vi "Image Difference RT Driver VI.vi"(10 "Device Outputs FIFO":refnum<k33>, 11 "Device Reference":T1 format="%.0x") -> ()   [LabVIEW 2012, in "Image Difference Custom Device.lvlib"]
uses:
  Image Difference Custom Device.lvlib
  <vilib>/NI Veristand/Custom Device API/Custom Device Item Ref.ctl
  <vilib>/NI Veristand/Custom Device API/Custom Device Channel Type.ctl
  <vilib>/NI Veristand/Custom Device API/Custom Device API.lvlib
  <vilib>/NI Veristand/Custom Device Tools/Custom Device Utility Library/Custom Device Utility Library.lvlib
  <vilib>/vision/driver/NI_Vision_Acquisition_Software.lvlib
panel:
  in  "Status Notifier":refnum<notifier>
  # "Custom Device Template\nv1.0"
  # "Use this template as a starting point for creating a custom device code module. The input controls shown here are specially named controls that the system will use to provide the device loop with data. The controls are not required for the device loop to run. For instance, if the device doesn't produce any output data, then you don't need the Device Outputs FIFO control. If you do use these controls, however, they need to have these exact names to be functional."
  # "The optional status notifier element is used to notify the RT engine of the last state of the custom device, and to indicate the device has completed execution. If this control is not used, a default No Error value is returned to the system when the device finishes execution.\n\nNote: This error state is not checked until the system shuts down. Use an output status channel to send more immediate status values to the system."
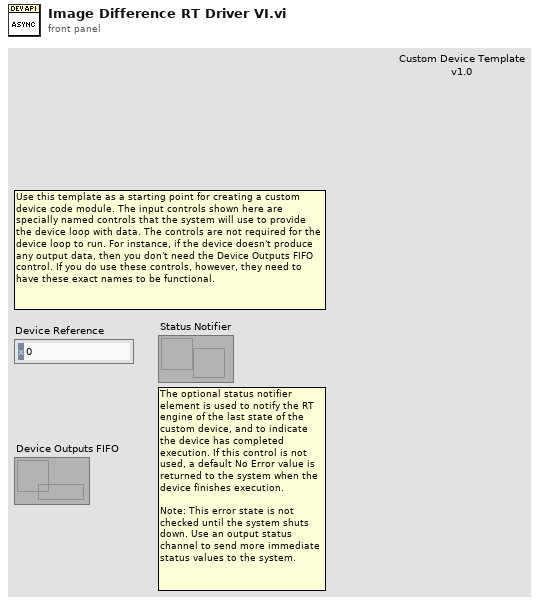
[diagram p1: front panel]
types:
  T1 = typedef "Custom Device API.lvlib/Custom Device Item Ref.ctl" = u64
  T2 = typedef "Custom Device API.lvlib/Custom Device Channel Type.ctl" = enum16{"Input", "Output"}
  T3 = typedef "IMAQdx.ctl" = refnum<k21>
  T4 = typedef "IMAQ Image.ctl" = refnum<image>
  T5 = typedef "Image Difference Custom Device.lvlib/Image Difference Info.ctl" = cluster{"ImgSub":T4, "SubDst":T4, "ImgMask":T4}
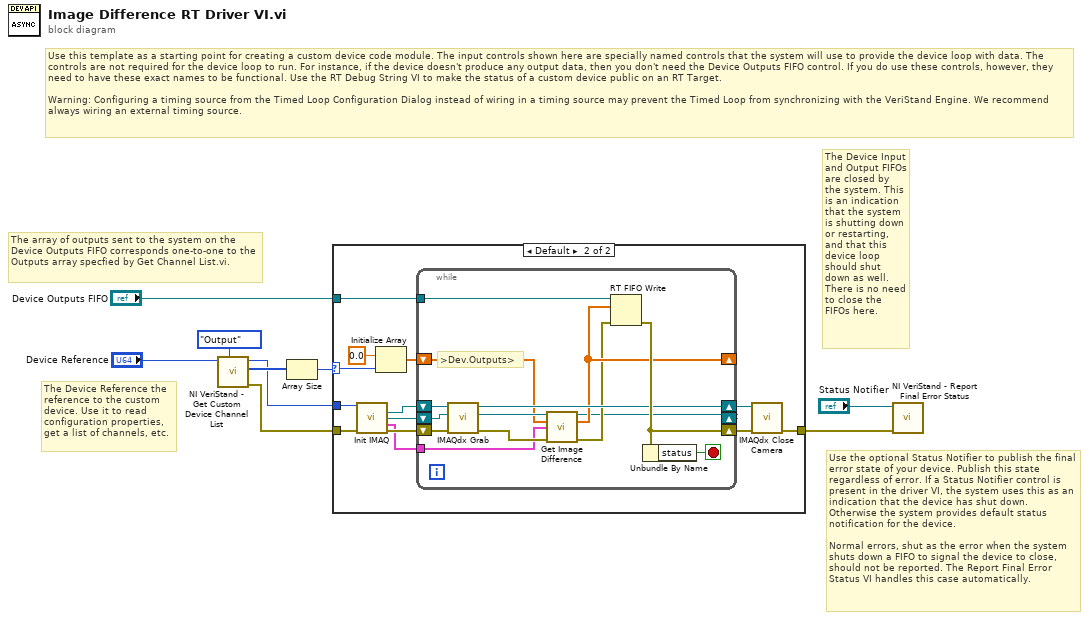
[diagram p0: block diagram]
diagram:
  # "Use the optional Status Notifier to publish the final error state of your device. Publish this state regardless of error. If a Status Notifier control is present in the driver VI, the system uses this as an indication that the device has shut down. Otherwise the system provides default status notification for the device.\n\nNormal errors, shut as the error when the system shuts down a FIFO to signal the device to close, should not be reported. The Report Final Error Status VI handles this case automatically."
  # "The Device Input and Output FIFOs are closed by the system. This is an indication that the system is shutting down or restarting, and that this device loop should shut down as well. There is no need to close the FIFOs here."
  # "The array of outputs sent to the system on the Device Outputs FIFO corresponds one-to-one to the Outputs array specfied by Get Channel List.vi."
  # "The Device Reference the reference to the custom device. Use it to read configuration properties, get a list of channels, etc."
  # "Use this template as a starting point for creating a custom device code module. The input controls shown here are specially named controls that the system will use to provide the device loop with data. The controls are not required for the device loop to run. For instance, if the device doesn't produce any output data, then you don't need the Device Outputs FIFO control. If you do use these controls, however, they need to have these exact names to be functional. Use the RT Debug String VI to make the status of a custom device public on an RT Target.\n\nWarning: Configuring a timing source from the Timed Loop Configuration Dialog instead of wiring in a timing source may prevent the Timed Loop from synchronizing with the VeriStand Engine. We recommend always wiring an external timing source."
  n1 = call <vilib>:"NI VeriStand - Get Custom Device Channel List.vi"("Channel Type"=Custom_Device_Channel_Type."Output", "Device Ref in"="Device Reference") -> ("error out"=w4:errorcluster, "Specified Channel Ref List"=w7:T1[], "Device Ref out"=w1:T1)  [unwired: 1 in, 6 out]
  n2 = Array Size(array=w7) -> (size(s)=w2:i32)
  n3 = case shown="Default" w2 {
    selector: w2 -> [_ w20]
    tunnel: "Device Outputs FIFO" -> [_ w23]
    tunnel: [w10 w13] -> w5
    tunnel: w4 -> [w10 w19]
    tunnel: w1 -> [_ w17]
    frame 0 {
    }
    frame Default {
      n4 = call "Init IMAQ.vi"("Custom Device In"=w17, "error in (no error)"=w19) -> ("Camera Session"=w16:T3, "Acquisition Image"=w15:T4, "Image Difference"=w11:T5, "error out"=w18:errorcluster)  [unwired: 9 in, 1 out]
      n5 = Initialize Array(0.0 ("element"), w20) -> (w21:dbl[])
      n6 = while {
        shift-right: [w36] -> w14
        shift-left: w18 -> [w34]
        shift-right: [w28] -> _
        shift-left: w21 -> [w29]
        tunnel: w23 -> [w37]
        tunnel: w11 -> [w24]
        shift-right: [w31] -> w12
        shift-left: w16 -> [w33]
        shift-right: [w25] -> _
        shift-left: w15 -> [w32]
        stop <- w35 stop-if-true
        # ">Dev.Outputs>"
        n7 = call <vilib>:"IMAQdx Grab.vi"("error in"=w34, "Image In"=w32, "Session In"=w33) -> ("error out"=w27:errorcluster, "Image Out"=w30:T4, "Session Out"=w31:T3)  [unwired: 1 in, 5 out]
        n8 = call "Get Image Difference.vi"("Acquisition Image In"=w30, "Channel Array In"=w29, "Image Difference Buffers"=w24, "error in (no error)"=w27) -> ("Acquisition Image Out"=w25:T4, "Channel Array Out"=w28:dbl[], "error out"=w26:errorcluster)  [unwired: 9 in]
        n9 = RT FIFO Write(0:w37, 1:w28, 3:w26) -> (11:w36:errorcluster)  [unwired: 1 in, 4 out]
        n10 = Unbundle By Name(w36) -> ("status"=w35:bool)
      }
      n11 = call <vilib>:"IMAQdx Close Camera.vi"("error in"=w14, "Session In"=w12) -> ("error out"=w13:errorcluster)  [unwired: 9 in]
    }
  }
  n12 = call <vilib>:"NI VeriStand - Report Final Error Status.vi"("error in (no error)"=w5, "Status Notifier"="Status Notifier") -> ()  [unwired: 1 in, 9 out]
